vi "adjust_plot_area_size.vi"(8 "error in":errorcluster, 10 "Draw Area Size":T1, 11 "ref":refnum<vi>) -> (0 "error out":errorcluster, 2 "final_width":u32, 3 "final_height":u32)   [LabVIEW 2017]
uses:
  <vilib>/Utility/miscctls.llb/LVBoundsTypeDef.ctl
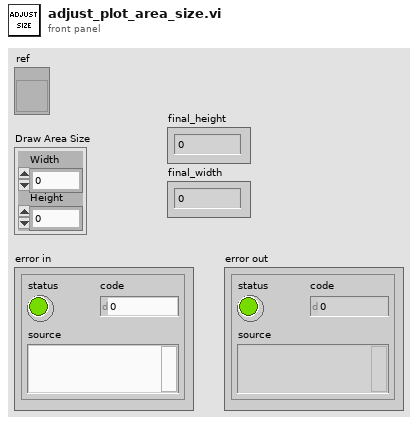
[diagram p1: front panel]
types:
  T1 = typedef "LVBoundsTypeDef.ctl" = cluster{"Width":u32, "Height":u32}
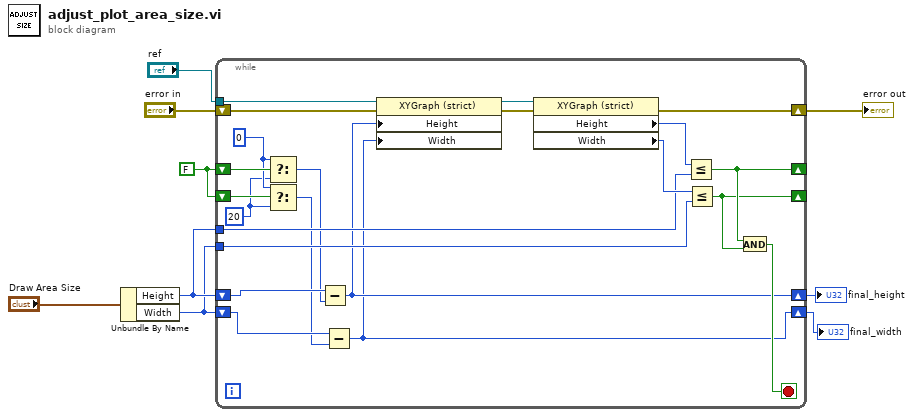
[diagram p0: block diagram]
diagram:
  w1 = FALSE
  n1 = Unbundle By Name("Draw Area Size") -> ("Height"=w8:u32, "Width"=w7:u32)
  n2 = while {
    shift-right: [w24] -> w9
    shift-left: "error in" -> [w31]
    shift-right: [w21] -> w3
    shift-left: w8 -> [w23]
    shift-right: [w20] -> w2
    shift-left: w7 -> [w22]
    tunnel: w7 -> [w28]
    tunnel: w8 -> [w26]
    tunnel: "ref" -> [w19]
    shift-right: [w17] -> _
    shift-left: w1 -> [w15]
    shift-right: [w16] -> _
    shift-left: w1 -> [w14]
    stop <- w25 stop-if-true
    w12 = u32 20 ("y")
    w13 = u32 0 ("y")
    n3 = Select(t=w13, s=w15, f=w12) -> (s? t:f=w10:u32)
    n4 = Select(t=w13, s=w14, f=w12) -> (s? t:f=w11:u32)
    n5 = Subtract(x=w23, y=w10) -> (x-y=w21:u32)
    n6 = Subtract(x=w22, y=w11) -> (x-y=w20:u32)
    n7 = property on="Property Node" class="XYGraph (strict)"(reference=w19, error in=w31, "Height"=w21, "Width"=w20) -> (reference out=w18:refnum<vi>, error out=w30:errorcluster)
    n8 = property on="Property Node" class="XYGraph (strict)"(reference=w18, error in=w30) -> (error out=w24:errorcluster, "Height"=w27:u32, "Width"=w29:u32)  [unwired: 1 out]
    n9 = Less Or Equal?(x=w27, y=w26) -> (x <= y?=w17:bool)
    n10 = Less Or Equal?(x=w29, y=w28) -> (x <= y?=w16:bool)
    n11 = And(x=w17, y=w16) -> (x .and. y?=w25:bool)
  }
  "error out" <- w9
  "final_height" <- w3
  "final_width" <- w2
